vi "AddPassed.vi"(8 "error in (no error)":errorcluster, 10 "TestCase":refnum<class "TestCase.lvclass">, 11 "EventTestListener in":refnum<class "EventTestListener.lvclass">) -> (0 "error out":errorcluster, 3 "EventTestListener out":refnum<class "EventTestListener.lvclass">)   [LabVIEW 2019, in "TestExplorer.lvlib" / "EventTestListener.lvclass"]
doc: "A test passed."
uses:
  EventTestListener.lvclass
  TestCase/TestCase/TestCase.lvclass
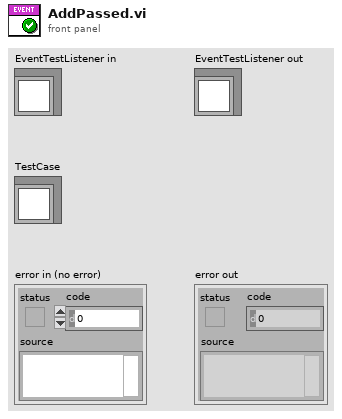
[diagram p1: front panel]
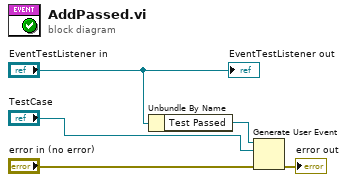
[diagram p0: block diagram]
diagram:
  n1 = Unbundle By Name("EventTestListener in") -> ("Test Passed"=w5:refnum<user-event>)
  n2 = Generate User Event(user event=w5, event data cluster="TestCase", error in="error in (no error)") -> (error out=→"error out":errorcluster)  [unwired: 1 in, 1 out]
  "EventTestListener out" <- "EventTestListener in"
